vi "Renew QDList In Multitable and Combox.vi"(8 "error in (no error)":errorcluster, 10 "Keyword(\"\")":string, 11 "ScriptsConfiguration in":refnum<class "ScriptSetting.lvclass">) -> (0 "error out":errorcluster, 3 "ScriptsConfiguration out":refnum<class "ScriptSetting.lvclass">)   [LabVIEW 2015, in "ScriptSetting.lvclass"]
uses:
  ScriptSetting.lvclass
  QDSearchList/QDDialogList.lvclass
  ScriptSetting.lvclass/ScriptSetting.ctl
  _Database/Implements/ScriptDatabase.lvclass
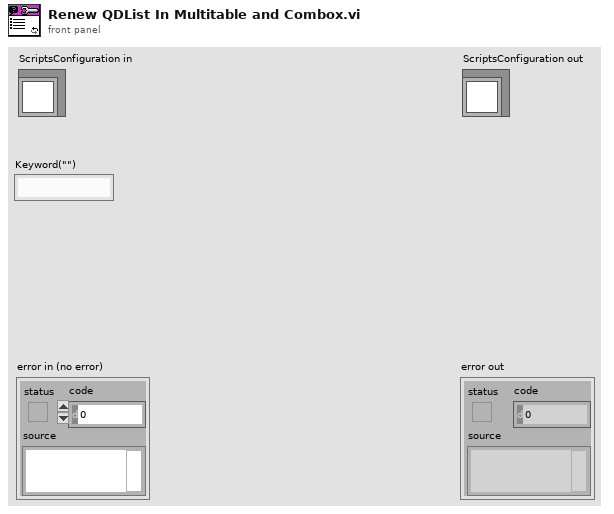
[diagram p1: front panel]
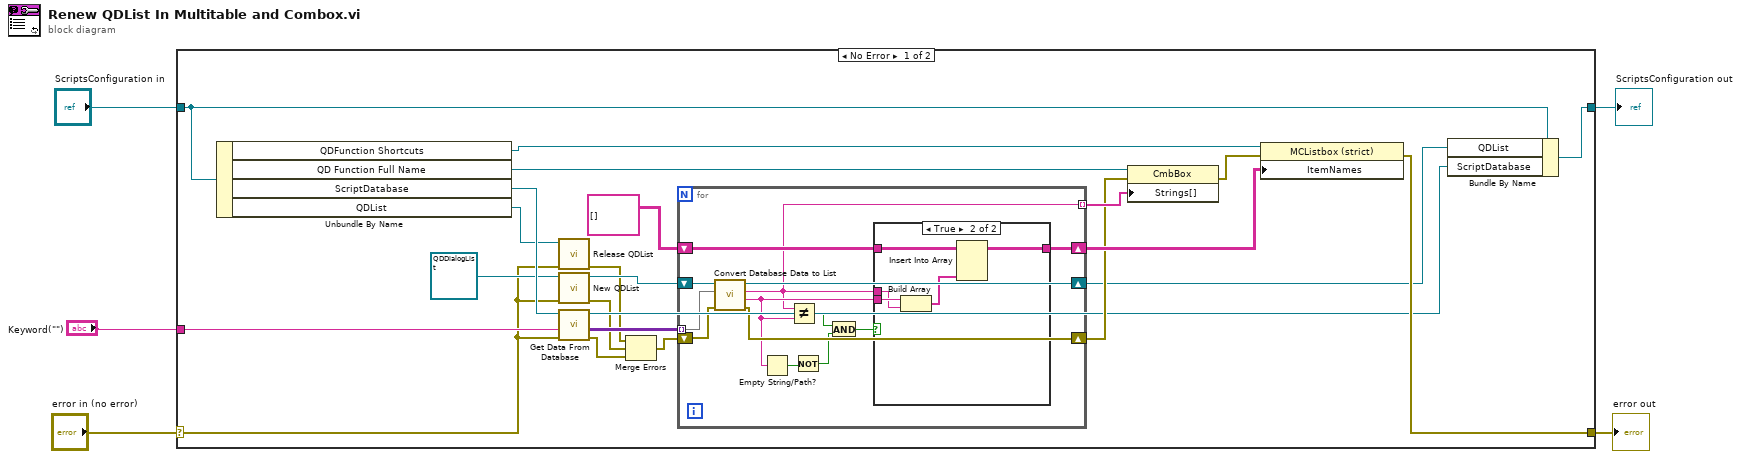
[diagram p0: block diagram]
diagram:
  n1 = case shown="No Error" "error in (no error)" {
    selector: "error in (no error)" -> [w7 w49]
    tunnel: [w19 w49] -> w4
    tunnel: [w16 w48] -> w2
    tunnel: "ScriptsConfiguration in" -> [w18 w48]
    tunnel: "Keyword(\"\")" -> [w15 _]
    frame No Error {
      n2 = Unbundle By Name(w18) -> ("QDFunction Shortcuts"=w23:refnum<vi>, "QD Function Full Name"=w25:refnum<vi>, "ScriptDatabase"=w28:refnum<class "ScriptDatabase.lvclass">, "QDList"=w8:refnum<class "QDDialogList.lvclass">)
      n3 = call "Release QDList.vi"("error in (no error)"=w7, "QDDialogList in"=w8) -> ("error out"=w6:errorcluster)  [unwired: 8 in, 1 out]
      n4 = call "New QDList.vi"("error in (no error)"=w7, "QDDialogList in"=refnum<class "QDDialogList.lvclass"> refnum ("NormalQDFunc out")) -> ("error out"=w10:errorcluster, "QDDialogList out"=w12:refnum<class "QDDialogList.lvclass">)  [unwired: 8 in]
      n5 = call "Get Data From Database.vi"("error in (no error)"=w7, "Keyword(\"\")"=w15, "ScriptDatabase in"=w28) -> ("error out"=w11:errorcluster, "recordset data"=w27:variant[][], "Database Out"=w14:refnum<class "ScriptDatabase.lvclass">)  [unwired: 6 in]
      n6 = Merge Errors(w6, w10, w11) -> (w9:errorcluster)
      n7 = for {
        tunnel: w27 -> [w40] mode=indexing
        shift-right: [w37] -> w22
        shift-left: string[][] [] -> [w38]
        tunnel: [w29] -> w24 mode=indexing
        shift-right: [w36] -> w21
        shift-left: w9 -> [w39]
        shift-right: [w35] -> w17
        shift-left: w12 -> [w41]
        n8 = call-dynamic "Convert Database Data to List.vi"("error in (no error)"=w39, "FetchedData"=w40, "NormalQDFunc in"=w41) -> ("error out"=w36:errorcluster, "QDFunction Acronym"=w34:string, "QDFunction Name"=w29:string, "NormalQDFunc out"=w35:refnum<class "QDDialogList.lvclass">)  [unwired: 5 in]
        n9 = Empty String/Path?(string/path=w34) -> (empty?=w31:bool)
        n10 = Not Equal?(x=w29, y=w34) -> (x != y?=w33:bool)
        n11 = Not(x=w31) -> (.not. x?=w30:bool)
        n12 = And(x=w33, y=w30) -> (x .and. y?=w32:bool)
        n13 = case shown="True" w32 {
          tunnel: w29 -> [_ w46]
          tunnel: w34 -> [_ w47]
          tunnel: w38 -> [w42 w45]
          tunnel: [w42 w43] -> w37
          frame False {
          }
          frame True {
            n14 = Build Array(w47, w46) -> (w44:string[])
            n15 = Insert Into Array(array=w45, new element=w44) -> (w43:string[][])  [unwired: 2 in]
          }
        }
      }
      n16 = property class="CmbBox"(reference=w25, error in=w21, "Strings[]"=w24) -> (error out=w20:errorcluster)  [unwired: 1 out]
      n17 = property class="MCListbox (strict)"(reference=w23, error in=w20, "ItemNames"=w22) -> (error out=w19:errorcluster)  [unwired: 1 out]
      n18 = Bundle By Name(cluster=w18, "QDList"=w17, "ScriptDatabase"=w14) -> (w16:refnum<class "ScriptSetting.lvclass">)
    }
    frame Error {
    }
  }
  "error out" <- w4
  "ScriptsConfiguration out" <- w2
